vi "Project_2(Main).vi"() -> ()   [LabVIEW 2023]
doc: "Project 2: Finite sate machine for loading and launching passengers in the Salvia Express"
uses:
  controls/enum defining states.ctl
  controls/Boolean output indicator.ctl
  controls/Boolean L E indictaor.ctl
  controls/enum defining DAQ actions.ctl
panel:
  out "L       E \nIndicator":T1 caption="L      E"
  out "Output\nIndicator":T2 caption="Z     Y     X"
  out "Reset?":bool
  out "Present State":T3
  in  "Stop Button":bool
  # "Salvia Express Passenger Control"
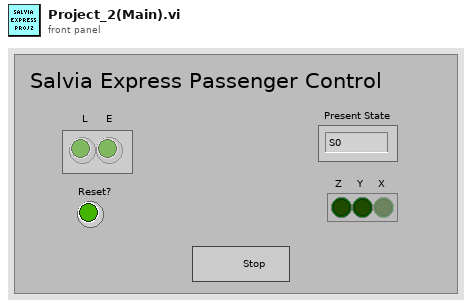
[diagram p1: front panel]
types:
  T1 = typedef "Boolean L E indictaor.ctl" = bool[]
  T2 = typedef "Boolean output indicator.ctl" = bool[]
  T3 = typedef "enum defining states.ctl" = enum16{"S0", "S1", "S2", "S3"}
  T4 = typedef "enum defining DAQ actions.ctl" = enum16{"Initialize DAQ", "Read L and  E  Commands", "Read R Command", "Write Outputs X, Y, and Z", "Release DAQ"}
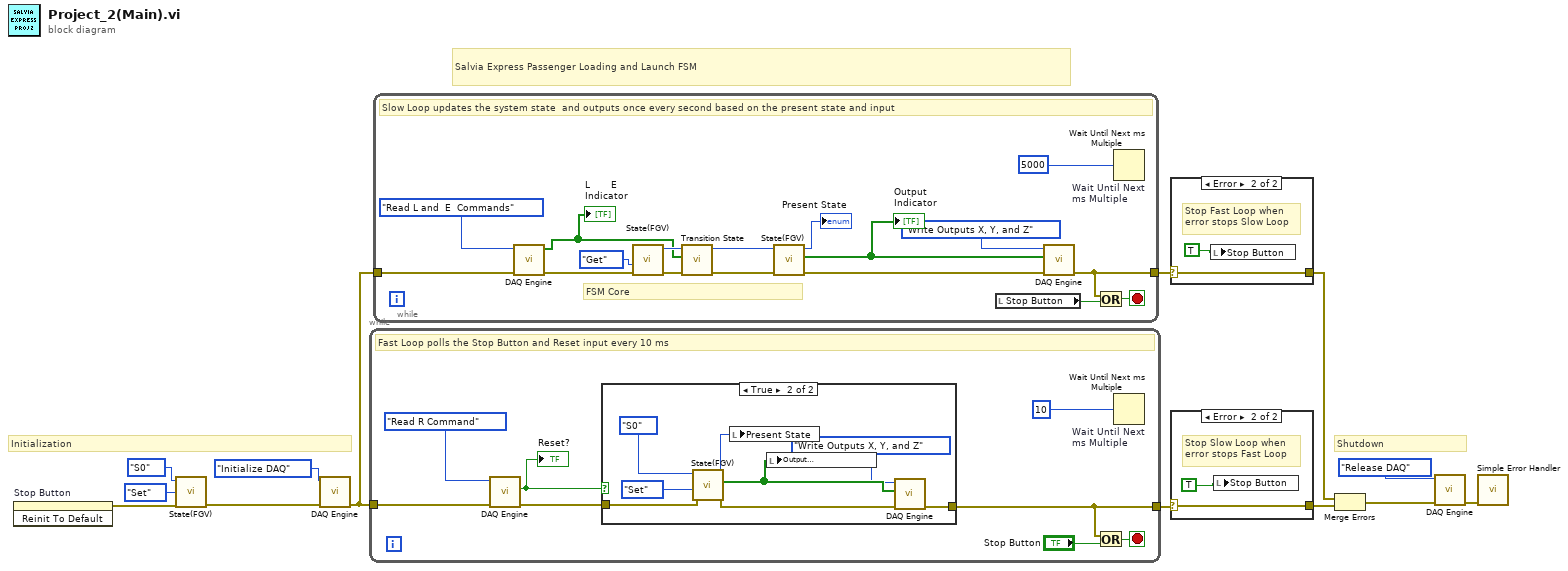
[diagram p0: block diagram]
diagram:
  # "Shutdown"
  # "Initialization"
  # "Salvia Express Passenger Loading and Launch FSM"
  n1 = invoke on="Stop Button" class="Bool (strict)" method="Reinit To Default"() -> (error out=w8:errorcluster)  [unwired: 3 in, 2 out]
  n2 = call "State(FGV).vi"("Error In"=w8, "Action"=enum16{"Set", "Get"}."Set", "input state"=enum_defining_states."S0" ("Input State")) -> ("Error Out"=w3:errorcluster)  [unwired: 6 in, 2 out]
  n3 = call "DAQ Engine.vi"("Error In"=w3, "DAQ Action"=enum_defining_DAQ_actions."Initialize DAQ") -> ("Error Out"=w10:errorcluster)  [unwired: 7 in, 2 out]
  n4 = while {
    tunnel: w10 -> [w21]
    tunnel: [w17] -> w6
    stop <- w19 stop-if-true
    # "Fast Loop polls the Stop Button and Reset input every 10 ms"
    n5 = call "DAQ Engine.vi"("Error In"=w21, "DAQ Action"=enum_defining_DAQ_actions."Read R Command") -> ("Error Out"=w20:errorcluster, "Reset ?"=w16:bool)  [unwired: 7 in, 1 out]
    "Reset?" <- w16
    n6 = case shown="True" w16 {
      tunnel: w20 -> [w22 w30]
      tunnel: [w22 w28] -> w17
      frame False {
      }
      frame True {
        n7 = call "State(FGV).vi"("Error In"=w30, "Action"=enum16{"Set", "Get"}."Set", "input state"=enum_defining_states."S0") -> ("Error Out"=w29:errorcluster, "Output \nIndicator"=w24:T2, "output state"=w27:T3)  [unwired: 6 in]
        n8 = local write "Present State"(w27) -> ()
        n9 = local write "Output\nIndicator"(w24) -> ()
        n10 = call "DAQ Engine.vi"("Error In"=w29, "Output \nIndicator"=w24, "DAQ Action"=enum_defining_DAQ_actions."Write Outputs X, Y, and Z") -> ("Error Out"=w28:errorcluster)  [unwired: 6 in, 2 out]
      }
    }
    n11 = Or(x=w17, y="Stop Button") -> (x .or. y?=w19:bool)
    n12 = Wait Until Next ms Multiple "Wait Until Next \nms Multiple"(millisecond multiple=u32 10) -> ()  [unwired: 1 out]
  }
  n13 = while {
    tunnel: w10 -> [w47]
    tunnel: [w39] -> w7
    stop <- w43 stop-if-true
    # "FSM Core"
    # "Slow Loop updates the system state  and outputs once every second based on the present state and input"
    n14 = call "DAQ Engine.vi"("Error In"=w47, "DAQ Action"=enum_defining_DAQ_actions."Read L and  E  Commands") -> ("Error Out"=w38:errorcluster, "L       E \nIndicator"=w34:T1)  [unwired: 7 in, 1 out]
    "L       E \nIndicator" <- w34
    n15 = call "State(FGV).vi"("Error In"=w38, "Action"=enum16{"Set", "Get"}."Get") -> ("Error Out"=w45:errorcluster, "output state"=w44:T3)  [unwired: 7 in, 1 out]
    n16 = call "Transition State.vi"("Error In"=w45, "L       E \nIndicator"=w34, "Present  State"=w44) -> ("Error Out"=w41:errorcluster, "Next State"=w42:T3)  [unwired: 7 in]
    n17 = call "State(FGV).vi"("Error In"=w41, "input state"=w42) -> ("Error Out"=w40:errorcluster, "Output \nIndicator"=w36:T2, "output state"=→"Present State":T3)  [unwired: 7 in]
    "Output\nIndicator" <- w36
    n18 = local read "Stop Button"() -> (w32:bool)
    n19 = call "DAQ Engine.vi"("Error In"=w40, "Output \nIndicator"=w36, "DAQ Action"=enum_defining_DAQ_actions."Write Outputs X, Y, and Z") -> ("Error Out"=w39:errorcluster)  [unwired: 6 in, 2 out]
    n20 = Or(x=w39, y=w32) -> (x .or. y?=w43:bool)
    n21 = Wait Until Next ms Multiple "Wait Until Next \nms Multiple"(millisecond multiple=u32 5000) -> ()  [unwired: 1 out]
  }
  n22 = case shown="Error" w7 {
    selector: w7 -> [w48 w50]
    tunnel: [w48 w50] -> w4
    frame No Error {
    }
    frame Error {
      # "Stop Fast Loop when\nerror stops Slow Loop"
      n23 = local write "Stop Button"(TRUE ("Stop Button")) -> ()
    }
  }
  n24 = case shown="Error" w6 {
    selector: w6 -> [w51 w53]
    tunnel: [w51 w53] -> w5
    frame No Error {
    }
    frame Error {
      # "Stop Slow Loop when\nerror stops Fast Loop"
      n25 = local write "Stop Button"(TRUE ("Stop Button")) -> ()
    }
  }
  n26 = Merge Errors(w4, w5) -> (w9:errorcluster)
  n27 = call "DAQ Engine.vi"("Error In"=w9, "DAQ Action"=enum_defining_DAQ_actions."Release DAQ") -> ("Error Out"=w11:errorcluster)  [unwired: 7 in, 2 out]
  n28 = call <vilib>:"Simple Error Handler.vi"("error in (no error)"=w11) -> ()  [unwired: 4 in, 5 out]
